vi "SaveZero.vi"(1 "error in":errorcluster, 2 "Zero value (in mm)":dbl) -> (0 "error out":errorcluster)   [LabVIEW 2013]
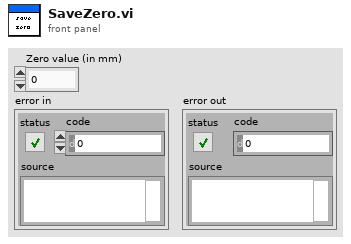
[diagram p1: front panel]
types:
  T1 = enum16{"open", "replace", "create", "open or create", "replace or create", "replace or create with confirmation"}
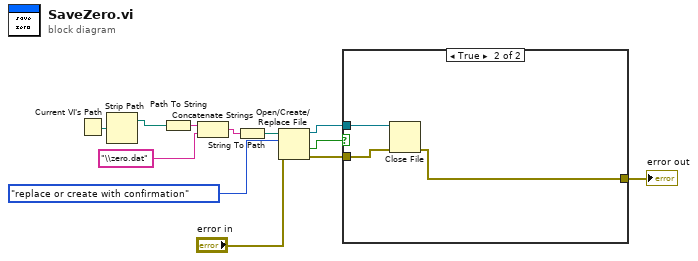
[diagram p0: block diagram]
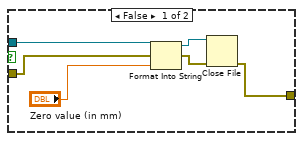
[diagram p2: hidden frame]
diagram:
  n1 = Current VI's Path() -> (path=w12:path)
  n2 = Strip Path(path=w12) -> (stripped path=w11:path)  [unwired: 1 out]
  n3 = Path To String(path=w11) -> (string=w10:string)
  n4 = Concatenate Strings(w10, "\\zero.dat" ("chaîne")) -> (w9:string)
  n5 = String To Path(string=w9) -> (path=w8:path)
  n6 = Open/Create/Replace File(file path (use dialog)=w8, error in="error in", operation (0:open)=T1."replace or create with confirmation") -> (refnum out=w5:refnum<file>, cancelled=w6:bool, error out=w4:errorcluster)  [unwired: 3 in]
  n7 = case shown="True" w6 {
    tunnel: w5 -> [w18 w21]
    tunnel: w4 -> [w17 w20]
    tunnel: [w13 w19] -> w1
    frame False {
      n8 = Format Into String(initial string=w18, error in=w17, "Zero value (in mm)") -> (resulting string=w16:refnum<file>, error out=w15:errorcluster)  [unwired: 1 in]
      n9 = Close File(refnum=w16, error in=w15) -> (error out=w13:errorcluster)  [unwired: 1 out]
    }
    frame True {
      n10 = Close File(refnum=w21, error in=w20) -> (error out=w19:errorcluster)  [unwired: 1 out]
    }
  }
  "error out" <- w1
